vi "Main Test.vi"   [LabVIEW 2013, in "Table Manager.lvlib"]
uses:
  Table Manager.lvlib
  Table Manager/references.ctl
  <vilib>/NI/Configuration Framework/Node/StopEvent.ctl
  <vilib>/NI/Configuration Framework/Node/RefreshUIEvent.ctl
  <vilib>/NI/Configuration Framework/Node/CacheState.ctl
  <vilib>/NI/Configuration Framework/Node/NodeChangeEvent.ctl
  <vilib>/NI/Configuration Framework/Node/NodeRef.ctl
  <vilib>/NI/Configuration Framework/Node/NISE_CEF_Node.lvclass
  <vilib>/NI/Tag Bus Data Framework/control module/editor node/channel action event.ctl
  <vilib>/NI/Tag Bus Data Framework/control module/editor node/dialog output action.ctl
  <vilib>/NI/Tag Bus Module Framework/channel/TBM channel.lvclass
  <vilib>/NI/Tag Bus/tag/tag descriptor.lvclass
  <vilib>/NI/AMC/Message Queue.ctl
  <vilib>/NI/AMC/Message.ctl
  <vilib>/NI/Tools/Keyed Array/KeyedArray.ctl
  <vilib>/NI/Configuration Framework/Node/UserEventRef.ctl
  <vilib>/NI/Configuration Framework/Controls/EventCluster.ctl
  Table Manager/object ref.ctl
  <vilib>/NI/Tag Bus Data Framework/Configuration Editor/Classes/Engine Parent/Engine Parent Editor Node.lvclass
  <vilib>/NI/Tag Bus Data Framework/Configuration Editor/Classes/Module editor node/module editor node.lvclass
  Column/Column Descriptor.ctl
  Column/Column Type.ctl
  Table Manager/Call Back Ref Type Def.ctl
  <vilib>/NI/Tag Bus/tag/Data Type.ctl
  Listbox/Multi Column Listbox.lvclass
  Data Grid/Data Grid.lvclass
  <vilib>/NI/Tag Bus Data Framework/control module/editor node/control module editor.lvclass
  <vilib>/NI/Tools/Keyed Array/Tools_KeyedArray.lvlib
  <vilib>/NI/AMC/AMC.lvlib
  <vilib>/NI/Configuration Framework/NISE_CEF_TreeControl.lvlib
  Table Manager/Table Manager.lvclass
  Column/Column.lvclass
types:
  T1 = typedef "Table Manager.lvlib/Column.lvclass/Column Descriptor.ctl" = cluster{"name":string, "caption":string, "Column Type":T2, "Params":string, "AutoSizeMode":i32, "FillWeight":sgl, "MinWidth":u32, "tooltip":string, "Enum Reference":refnum<vi>, "Channel suffix":string, "Read Only":bool, "Call Back VI":T3, "DT Dependency":i32, "name dependency":i32, "data type":T4}
  T2 = typedef "Table Manager.lvlib/Column.lvclass/Column Type.ctl" = enum16{"String", "Mapping", "Channel Name", "Tag", "Enum", "Data Type", "Numeric"}
  T3 = typedef "Table Manager.lvlib/Table Manager.lvclass/Call Back Ref Type Def.ctl" = refnum<vi>
  T4 = typedef "tag bus.lvlib/tag descriptor.lvclass/Data Type.ctl" = enum16{"Double", "Single", "I64", "I32", "I16", "I8", "U64", "U32", "U16", "U8", "Boolean", "String", "Array of Double", "Array of Single", "Array of I64", "Array of I32", "Array of I16", "Array of I8", "Array of U64", "Array of U32", "Array of U16", "Array of U8", "Array of Boolean", "Array of String"}
  T5 = typedef "Table Manager.lvlib/Table Manager.lvclass/object ref.ctl" = cluster{"engine":refnum<data-value>, "Node Ref":refnum<data-value>}
  T6 = typedef "Table Manager.lvlib/Table Manager.lvclass/references.ctl" = cluster{"stop event":T7, "refresh UI":T8, "cache state":T9, "node change":T10, "user event out":refnum<user-event>, "main queue":T11, "user event":T12}
  T7 = typedef "NISE_CEF_Node.lvclass/StopEvent.ctl" = refnum<user-event>
  T8 = typedef "NISE_CEF_Node.lvclass/RefreshUIEvent.ctl" = refnum<user-event>
  T9 = typedef "NISE_CEF_Node.lvclass/CacheState.ctl" = refnum<user-event>
  T10 = typedef "NISE_CEF_Node.lvclass/NodeChangeEvent.ctl" = refnum<user-event>
  T11 = typedef "AMC.lvlib/Message Queue.ctl" = refnum<queue>
  T12 = typedef "NISE_CEF_Node.lvclass/UserEventRef.ctl" = refnum<user-event>
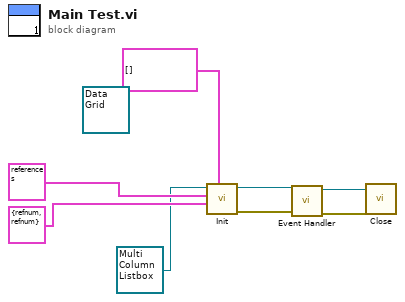
[diagram p0: block diagram]
diagram:
  (unwired) refnum<class "Data Grid.lvclass"> refnum ("Table Manager.lvlib:Data Grid.lvclass")
  n1 = call-dynamic "Init.vi"("Column Definitions"=T1[] [], "object refs"=T5 {"engine"=refnum, "Node Ref"=refnum}, "References in"=T6 {"stop event"=refnum, "refresh UI"=refnum, "cache state"=refnum, "node change"=refnum, "user event out"=refnum, "main queue"=refnum, "user event"=refnum}, "Multi Column Listbox in"=refnum<class "Multi Column Listbox.lvclass"> refnum ("Table Manager.lvlib:Listbox.lvclass")) -> ("error out"=w3:errorcluster, "Multi Column Listbox out"=w8:refnum<class "Multi Column Listbox.lvclass">)  [unwired: 5 in, 1 out]
  n2 = call-dynamic "Event Handler.vi"("error in"=w3, "Listbox in"=w8) -> ("error out"=w2:errorcluster, "Listbox out"=w7:refnum<class "Multi Column Listbox.lvclass">)  [unwired: 8 in]
  n3 = call-dynamic "Close.vi"("error in (no error)"=w2, "Multi Column Listbox in"=w7) -> ()  [unwired: 8 in, 2 out]
